vi "Null Py Object Refnum.vi"() -> (0 "Null Python Object Refnum":T1)   [LabVIEW 2020, in "G-Embedded-Python-Interpreter-Toolkit.lvlib"]
uses:
  G-Embedded-Python-Interpreter-Toolkit.lvlib
  Python Object Reference.ctl
  Python Object Type.ctl
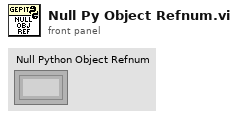
[diagram p1: front panel]
types:
  T1 = typedef "G-Embedded-Python-Interpreter-Toolkit.lvlib/Python Object Reference.ctl" = refnum<k1>
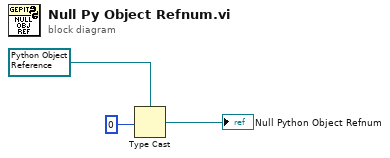
[diagram p0: block diagram]
diagram:
  w2 = T1 refnum items=["PObj"] ("Python Object Refnum")
  n1 = Type Cast(type=w2, x=u32 0) -> (*(type *) &x=→"Null Python Object Refnum":T1)
